vi "GT Pvt Status.vi"(6 "count":i16, 7 "pTime":dbl, 8 "error in (no error)":errorcluster caption="错误输入（无错误）", 9 "pTableId":i16, 10 "profile":i16, 11 "cardNum":i16) -> (0 "error out":errorcluster caption="错误输出", 1 "pTableId out":i16, 3 "function return":i16, 5 "pTime out":dbl)   [LabVIEW 2014, in "gts.lvlib"]
doc: "GT_API GT_PvtStatus(short cardNum,short profile,short *pTableId,double *pTime,short count=1);"
uses:
  gts.lvlib
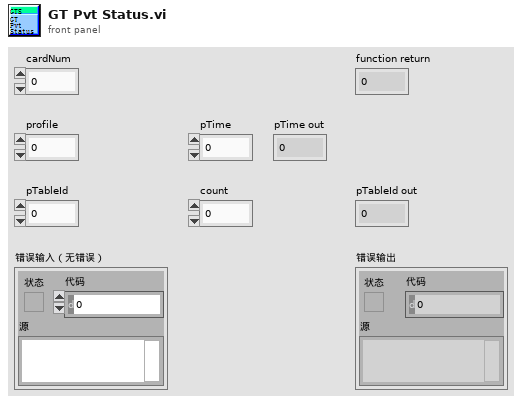
[diagram p1: front panel]
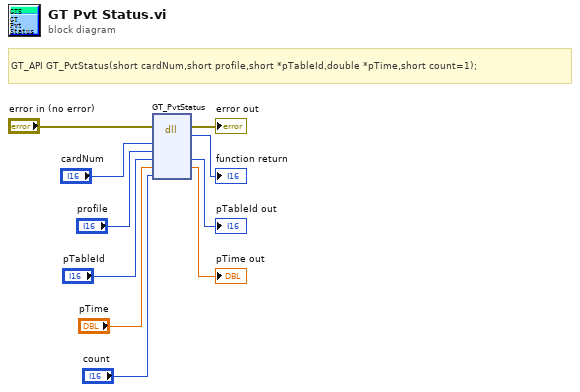
[diagram p0: block diagram]
diagram:
  # "GT_API GT_PvtStatus(short cardNum,short profile,short *pTableId,double *pTime,short count=1);"
  n1 = dll-call lib="PTH2habs D固高科技资料GTS控制卡GTS卡18年上半年资料dllVC32bit\nmulti_cardgts.*" fn="GT_PvtStatus"(error in="error in (no error)", "cardNum"="cardNum", "profile"="profile", "pTableId"="pTableId", "pTime"="pTime", "count"="count") -> (error out=→"error out":errorcluster, →"function return":i16, "pTableId"=→"pTableId out":i16, "pTime"=→"pTime out":dbl)  [unwired: 5 in, 1 out]
